vi "Scan PZT V parameter.vi"(11 "字符串":string) -> (0 "间隔":dbl=4.0, 1 "最小电压":dbl=-48.0, 2 "最大电压":dbl=148.0, 3 "零电压":dbl)   [LabVIEW 2019, in "nematic.lvlib"]
uses:
  nematic.lvlib
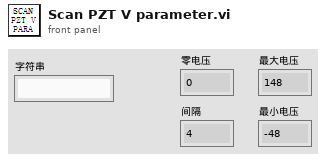
[diagram p1: front panel]
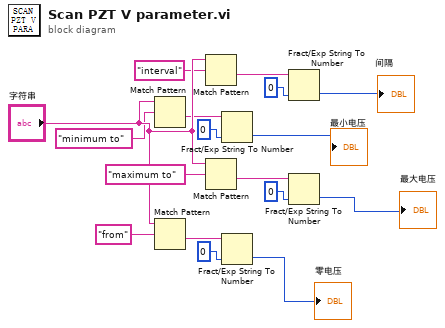
[diagram p0: block diagram]
diagram:
  n1 = Match Pattern(string="字符串", regular expression="minimum to" ("正则表达式")) -> (after substring=w6:string)  [unwired: 1 in, 3 out]
  n2 = Match Pattern(string="字符串", regular expression="from" ("正则表达式")) -> (after substring=w14:string)  [unwired: 1 in, 3 out]
  n3 = Match Pattern(string="字符串", regular expression="interval" ("正则表达式")) -> (after substring=w5:string)  [unwired: 1 in, 3 out]
  n4 = Match Pattern(string="字符串", regular expression="maximum to" ("正则表达式")) -> (after substring=w7:string)  [unwired: 1 in, 3 out]
  n5 = Fract/Exp String To Number(string=w6, default (0 dbl)=0) -> (number=→"最小电压":i32)  [unwired: 2 in, 1 out]
  n6 = Fract/Exp String To Number(string=w14, default (0 dbl)=0) -> (number=→"零电压":i32)  [unwired: 2 in, 1 out]
  n7 = Fract/Exp String To Number(string=w5, default (0 dbl)=0) -> (number=→"间隔":i32)  [unwired: 2 in, 1 out]
  n8 = Fract/Exp String To Number(string=w7, default (0 dbl)=0) -> (number=→"最大电压":i32)  [unwired: 2 in, 1 out]
